vi "Num to array.vi"(11 "Input array":u8[](array[numeric])) -> (3 "Bool array":bool[](array[boolean]))   [LabVIEW 2020, in "NI DAQ Aug 25.lvlib"]
uses:
  NI DAQ Aug 25.lvlib
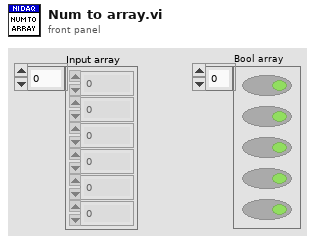
[diagram p1: front panel]
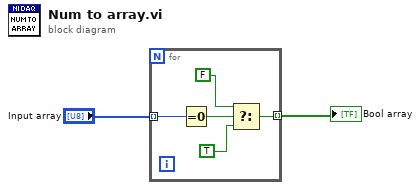
[diagram p0: block diagram]
diagram:
  n1 = for {
    tunnel: "Input array" -> [w7] mode=indexing
    tunnel: [w3] -> w1 mode=indexing
    n2 = Equal To 0?(x=w7) -> (x = 0?=w6:bool)
    n3 = Select(t=FALSE, s=w6, f=TRUE) -> (s? t:f=w3:bool)
  }
  "Bool array" <- w1
